vi "PictureToFXP.vi"(11 "Accessors:Picture":T1) -> (3 "Array":fxp<+,3,3>[](array[numeric]))   [LabVIEW 2019, in "RT_Game.lvlib" / "SpriteHandler.lvclass"]
uses:
  SpriteHandler.lvclass
  <vilib>/picture/picture.llb/imagedata.ctl
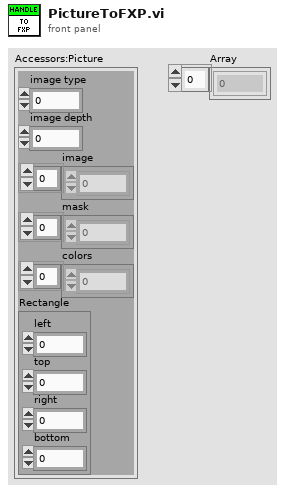
[diagram p1: front panel]
types:
  T1 = typedef "imagedata.ctl" = cluster{"image type":i32, "image depth":i32, "image":u8[], "mask":u8[], "colors":u32[], "Rectangle":cluster{"left":i16, "top":i16, "right":i16, "bottom":i16}}
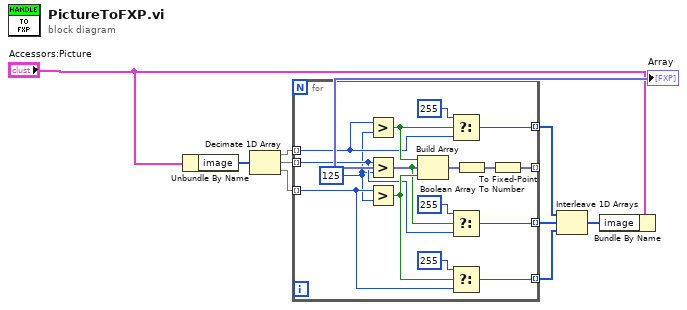
[diagram p0: block diagram]
diagram:
  n1 = Unbundle By Name("Accessors:Picture") -> ("image"=w7:u8[])
  n2 = Decimate 1D Array(w7) -> (w8:u8[], w9:u8[], w10:u8[])
  n3 = for {
    tunnel: w8 -> [w15] mode=indexing
    tunnel: w9 -> [w19] mode=indexing
    tunnel: w10 -> [w18] mode=indexing
    tunnel: [w24] -> w2 mode=indexing
    tunnel: [w13] -> w5 mode=indexing
    tunnel: [w12] -> w4 mode=indexing
    tunnel: [w11] -> w3 mode=indexing
    w14 = u8 125 ("y")
    n4 = Greater?(x=w15, y=w14) -> (0:w23:bool)
    n5 = Greater?(x=w19, y=w14) -> (0:w21:bool)
    n6 = Greater?(x=w18, y=w14) -> (0:w22:bool)
    n7 = Build Array(w23, w21, w22) -> (w26:bool[])
    n8 = Select(t=u8 255, s=w23, f=w15) -> (s? t:f=w13:u8)
    n9 = Select(t=u8 255, s=w21, f=w19) -> (s? t:f=w12:u8)
    n10 = Select(t=u8 255, s=w22, f=w18) -> (s? t:f=w11:u8)
    n11 = Boolean Array To Number(Boolean array=w26) -> (number=w25:u32)
    n12 = To Fixed-Point(number=w25) -> (fixed-point=w24:fxp<+,3,3>)  [unwired: 1 in]
  }
  "Array" <- w2
  n13 = Interleave 1D Arrays(w5, w4, w3) -> (w6:u8[])
  n14 = Bundle By Name(cluster="Accessors:Picture", "image"=w6) -> ()  [unwired: 1 out]
